vi "data_distributor.vi"(0 "Analog Data Array":T2[](array[typedef]), 1 "Pressure/Temperature/Mixture Properties Refnum":refnum<vi>, 2 "Measurements Data Refnum":refnum<vi>, 3 "Cluster 2":T1, 9 "Indicies":T3[](array[typedef]), 11 "error in":errorcluster, 12 "Diode ChartsRefnum":refnum<vi>, 13 "Vapor PID Refnum":refnum<vi>, 14 "Liquid PID Refnum":refnum<vi>) -> (15 "error out":errorcluster)   [LabVIEW 2017]
uses:
  Utility Sub VIs/pressure_temp_mixture.ctl
  Utility Sub VIs/pulse_generator_data.ctl
  Utility Sub VIs/diode_charts.ctl
  analog_data.ctl
  index_array_cluster.ctl
  Utility Sub VIs/valve_pid_control.ctl
panel:
  # "Pulse Gen"
  # "Test Section"
  # "Saturation\nPressure [Pa]"
  # "Saturation\nTemperature [C]"
  # "Pressure [Pa]"
  # "Temperature [C]"
  # "Liquid Tank"
  # "Separator"
  # "Liquid Inlet"
  # "Vapor Tank"
  # "Vapor Inlet"
  # "Test Section"
  # "Upper Dev Section"
  # "Lower Dev Section"
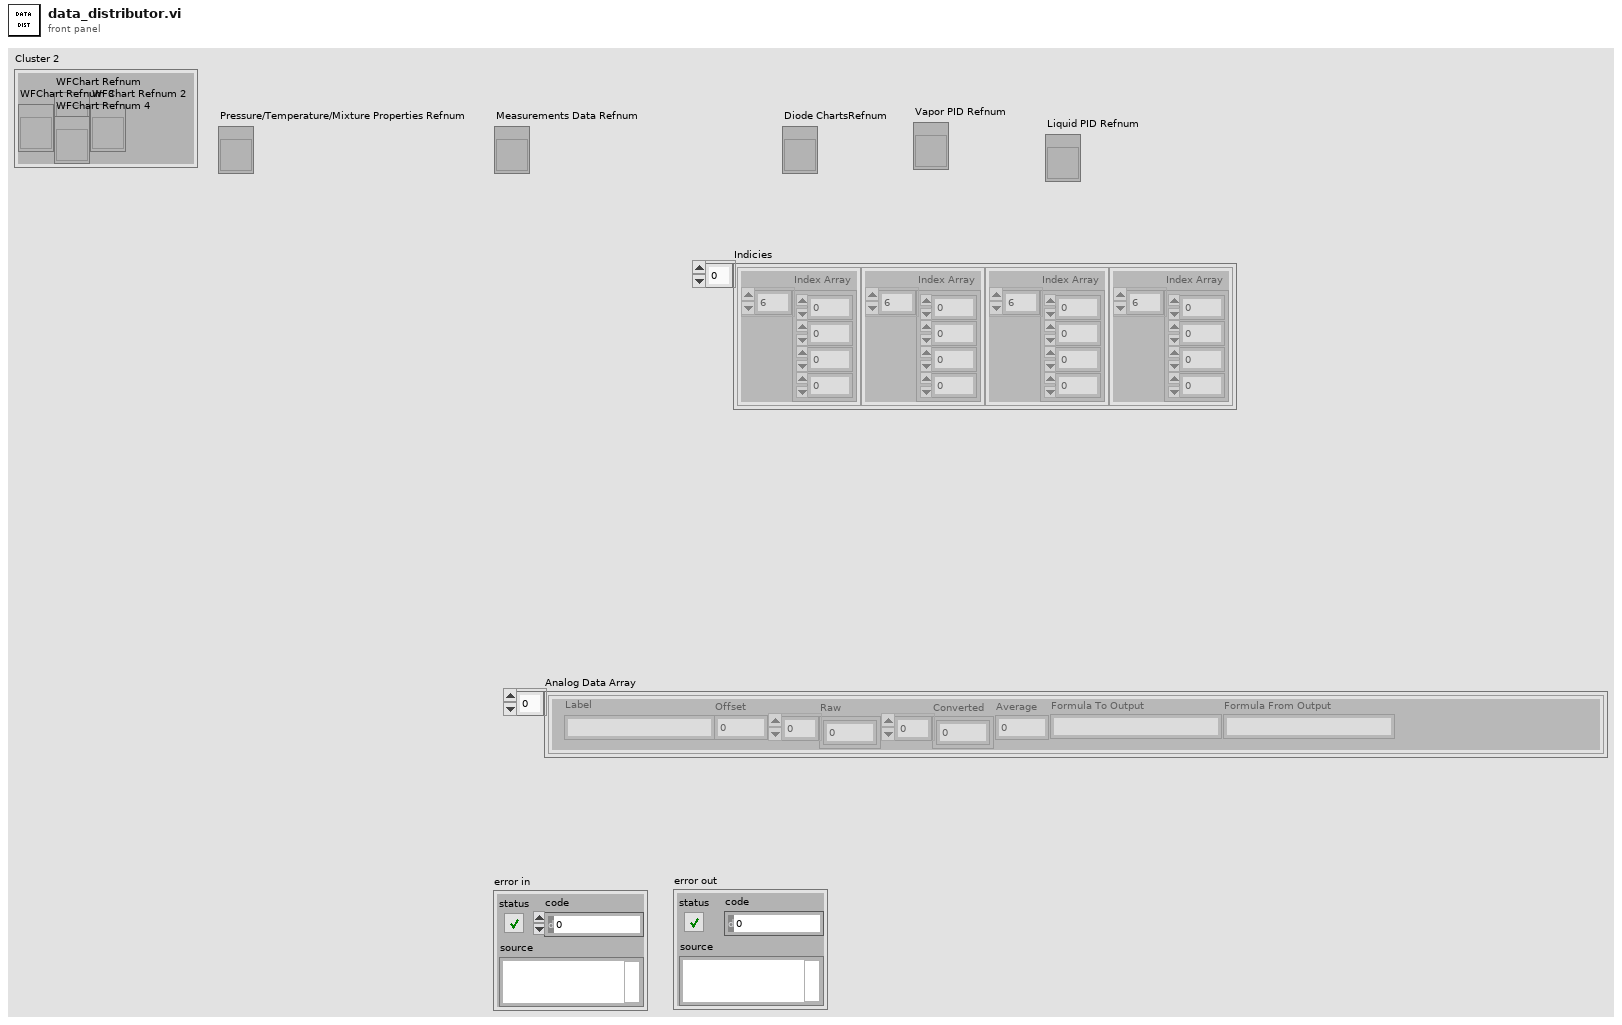
[diagram p1: front panel]
types:
  T1 = cluster{"WFChart Refnum":refnum<vi>, "WFChart Refnum 2":refnum<vi>, "WFChart Refnum 3":refnum<vi>, "WFChart Refnum 4":refnum<vi>}
  T2 = typedef "analog_data.ctl" = cluster{"Label":string, "Offset":dbl, "Raw":dbl[], "Converted":dbl[], "Average":dbl, "Formula To Output":string, "Formula From Output":string}
  T3 = typedef "index_array_cluster.ctl" = cluster{"Index Array":i32[]}
  T4 = cluster{"Mixing Tee dP":dbl, "PG inlet-Mixing Tee Abs Pressure":dbl, "PG inlet-Mixing Tee Temperature":dbl}
  T5 = typedef "pressure_temp_mixture.ctl" = cluster{"Line Densities\n[g/cm^3]":cluster{"Vapor Line":dbl, "Liquid Line":dbl}, "Mixture Properties":cluster{"Enthalpy":dbl, "Quality [-]":dbl}, "Component PTs":cluster{"Liquid Tank P":dbl, "Liquid Tank T":dbl, "Liquid Tank Sat P":dbl, "Liquid Tank Sat T":dbl, "Separator P":dbl, "Separator T":dbl, "Separator Sat P":dbl, "Separator Sat T":dbl, "Liquid Inlet P":dbl, "Liquid Inlet T":dbl, "Liquid Inlet Sat P":dbl, "Liquid Inlet Sat T":dbl, "Vapor Tank P":dbl, "Vapor Tank T":dbl, "Vapor Tank Sat P":dbl, "Vapor Tank Sat T":dbl, "Vapor Inlet P":dbl, "Vapor Inlet T":dbl, "Vapor Inlet Sat P":dbl, "Vapor Inlet Sat T":dbl, "Test Section P":dbl, "Test Section T":dbl, "Test Section Sat P":dbl, "Test Section Sat T":dbl, "Upper Dev Section P":dbl, "Upper Dev Section T":dbl, "Upper Dev Section Sat P":dbl, "Upper Dev Section Sat T":dbl, "Lower Dev Section P":dbl, "Lower Dev Section T":dbl, "Lower Dev Section Sat P":dbl, "Lower Dev Section Sat T":dbl}, "Ambient Pressure [Pa]":dbl, "Mixing Tee":cluster{"Venturi dP":dbl, "PGminiPressure":dbl, "PGminiTemperature":dbl}}
  T6 = cluster{"[0]":dbl, "[1]":dbl, "[2]":dbl, "[3]":dbl, "[4]":dbl, "[5]":dbl, "[6]":dbl, "[7]":dbl, "[8]":dbl, "[9]":dbl, "[10]":dbl, "[11]":dbl, "[12]":dbl, "[13]":dbl, "[14]":dbl, "[15]":dbl, "[16]":dbl, "[17]":dbl, "[18]":dbl, "[19]":dbl, "[20]":dbl, "[21]":dbl, "[22]":dbl, "[23]":dbl, "[24]":dbl, "[25]":dbl, "[26]":dbl, "[27]":dbl, "[28]":dbl, "[29]":dbl, "[30]":dbl, "[31]":dbl}
  T7 = cluster{"Mass Flow Rate [g/s]":dbl, "Mass Flow Rate [g/s]":dbl}
  T8 = cluster{"[0]":dbl, "[1]":dbl, "[2]":dbl, "[3]":dbl, "[4]":dbl, "[5]":dbl, "[6]":dbl, "[7]":dbl, "[8]":dbl, "[9]":dbl, "[10]":dbl, "[11]":dbl, "[12]":dbl, "[13]":dbl, "[14]":dbl, "[15]":dbl}
  T9 = typedef "valve_pid_control.ctl" = cluster{"Flow":cluster{"Flow rate [g/s]":dbl, "Line Density [g/cm^3]":dbl}, "Valve On/Off":bool, "PID Mode":bool, "PLC Calc Basis":bool, "Flow Set Point [g/s]":dbl, "Pump Output [%]":dbl, "Valve Open Voltage [V]":dbl, "Flow Setpoint Adrs":u16, "Pump Output Adrs":u16, "Manual Mode Request Adrs":u16, "Manual Mode Adrs":u16}
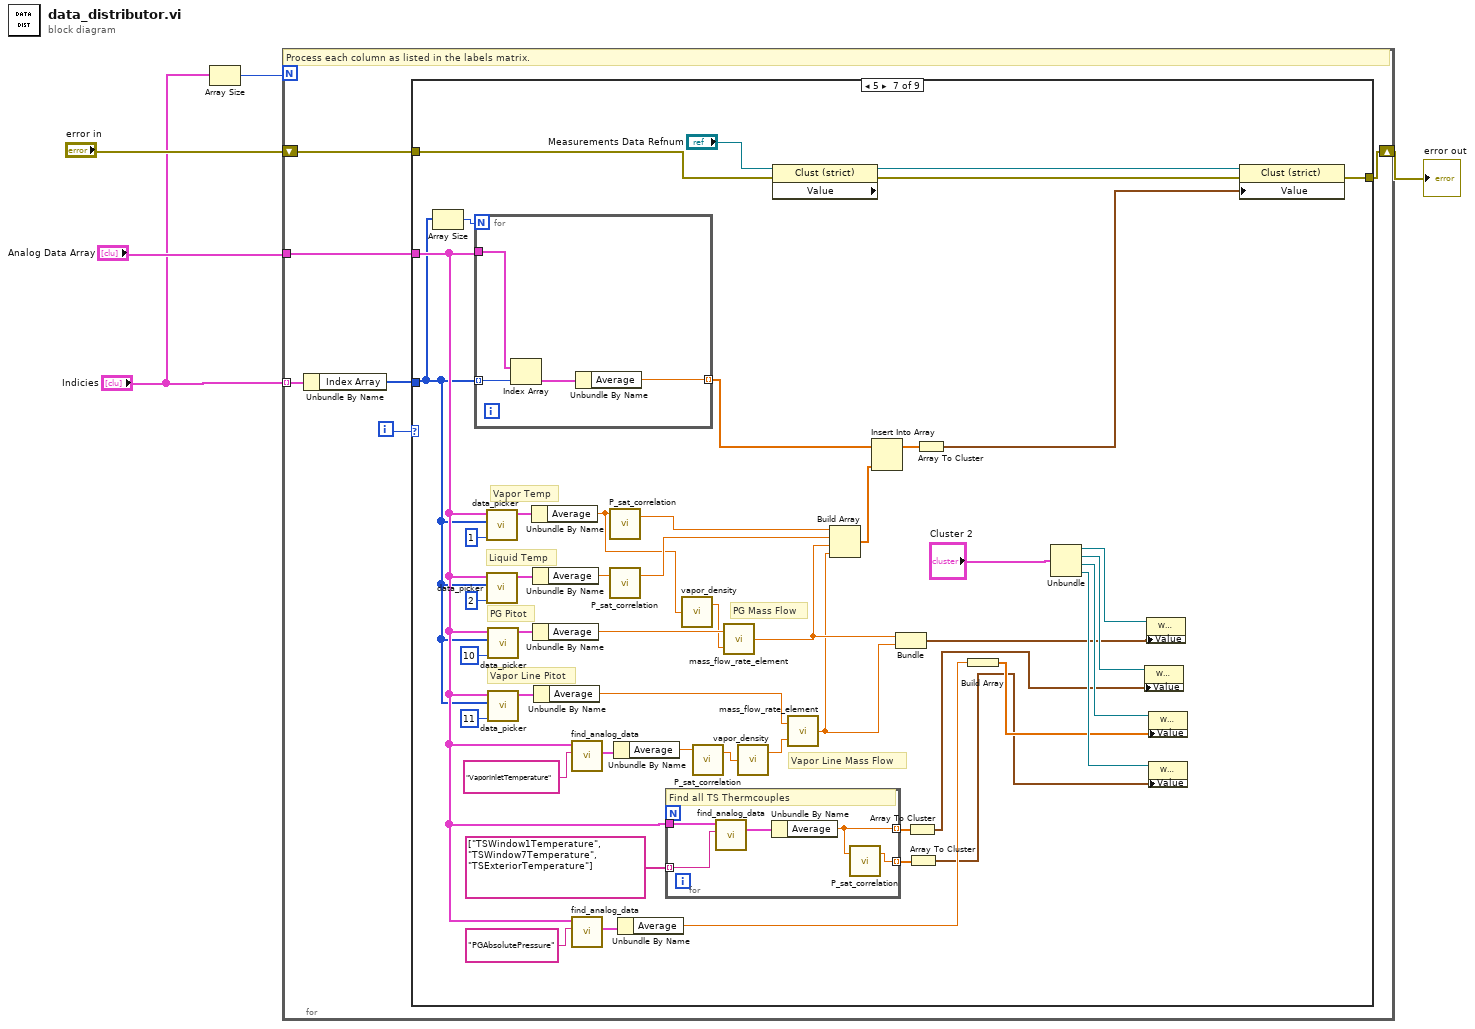
[diagram p0: block diagram]
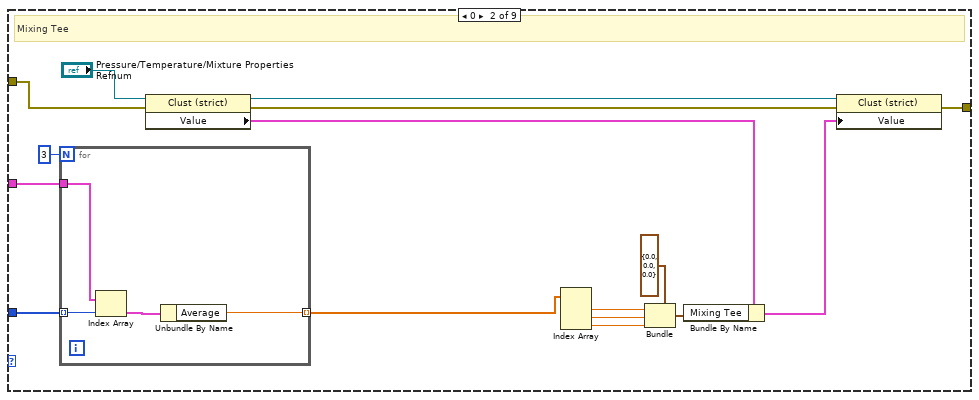
[diagram p3: hidden frame]
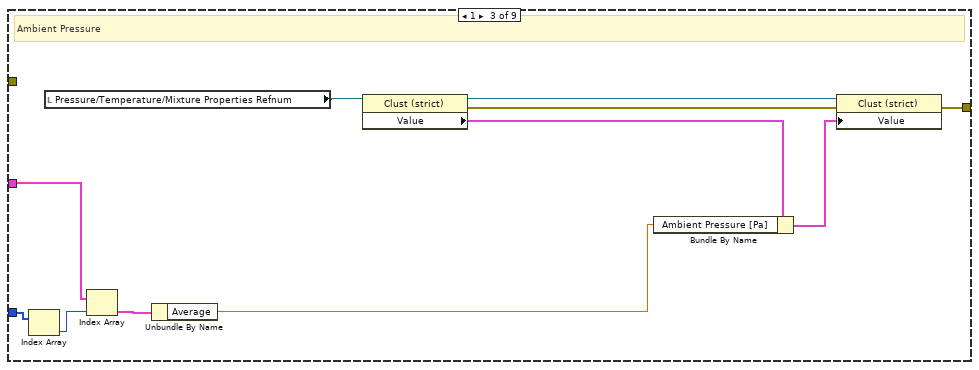
[diagram p4: hidden frame]
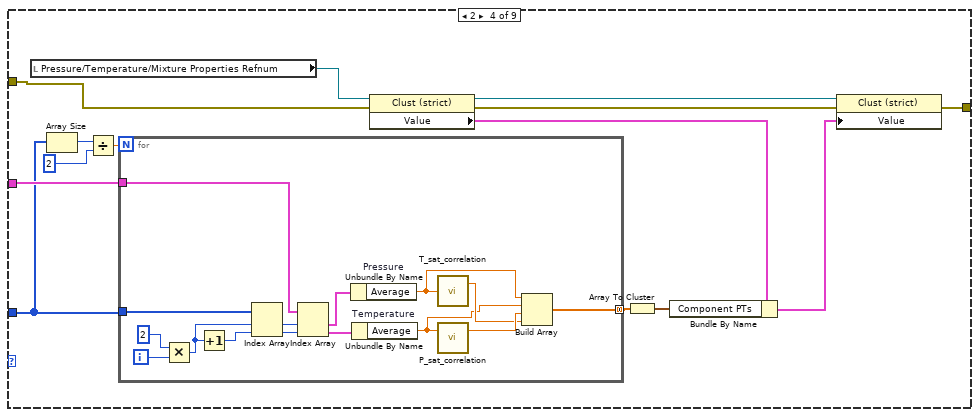
[diagram p5: hidden frame]
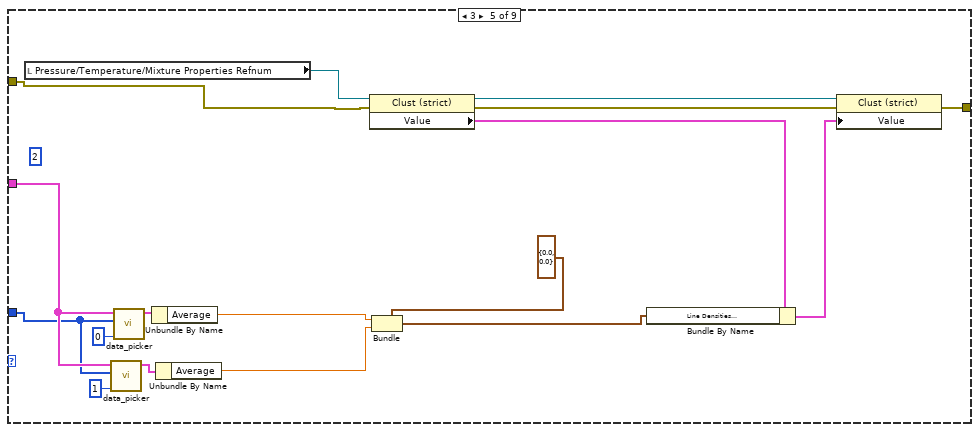
[diagram p6: hidden frame]
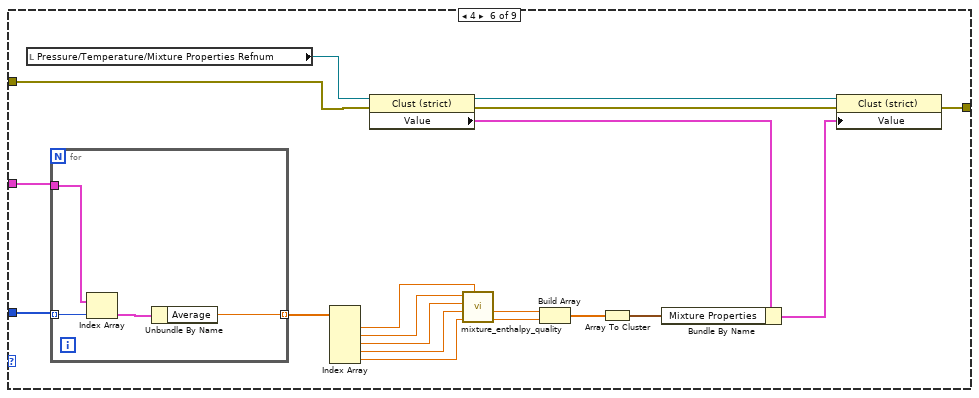
[diagram p7: hidden frame]
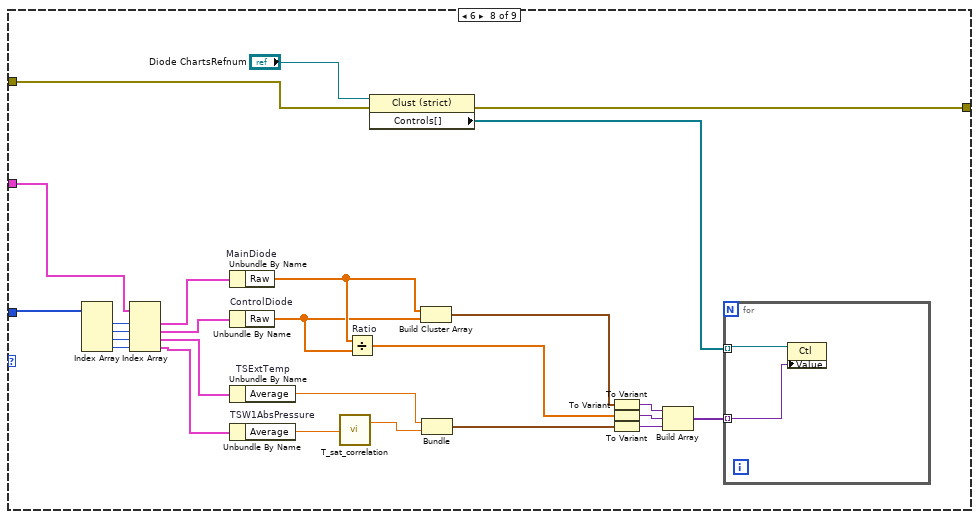
[diagram p8: hidden frame]
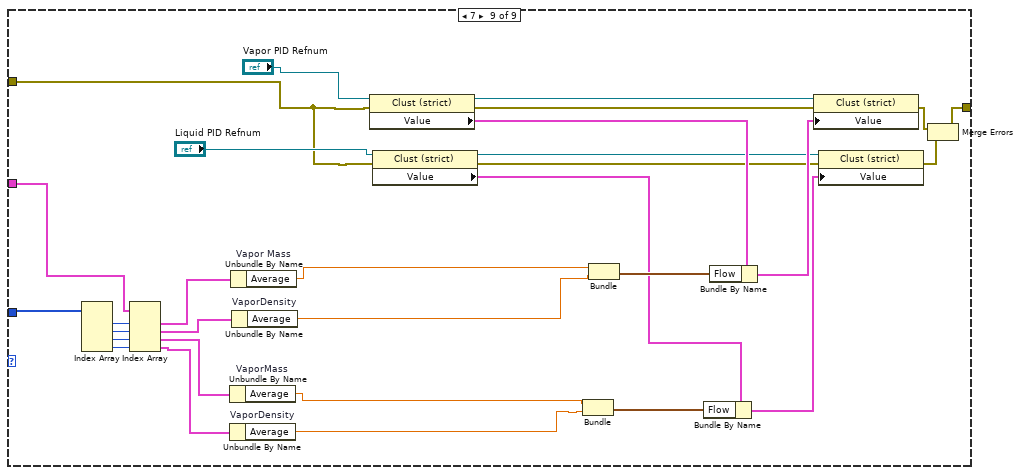
[diagram p9: hidden frame]
diagram:
  n1 = Array Size(array="Indicies") -> (size(s)=w4:i32)
  n2 = for {
    N: w4 -> [_]
    tunnel: "Analog Data Array" -> [w10]
    tunnel: "Indicies" -> [w6] mode=indexing
    shift-right: [w8] -> w5
    shift-left: "error in" -> [w9]
    i -> [w11]
    # "Process each column as listed in the labels matrix."
    n3 = Unbundle By Name(w6) -> ("Index Array"=w7:i32[])
    n4 = case shown="5" w11 {
      tunnel: w7 -> [_ w24 w34 w52 w79 w103 w122 w191 w228]
      tunnel: w10 -> [_ w23 w39 w53 w80 w104 w130 w189 w226]
      tunnel: w9 -> [w12 w20 _ w44 w84 w91 w124 w171 w200]
      tunnel: [w12 w22 w37 w46 w85 w92 w127 w173 w202] -> w8
      frame Default {
      }
      frame 0 {
        # "Mixing Tee"
        n5 = for {
          N: 3 -> [_]
          tunnel: w24 -> [w32] mode=indexing
          tunnel: w23 -> [w31]
          tunnel: [w29] -> w17 mode=indexing
          n6 = Index Array(array=w31, index=w32) -> (element=w30:T2)
          n7 = Unbundle By Name(w30) -> ("Average"=w29:dbl)
        }
        n8 = property class="Clust (strict)"(reference="Pressure/Temperature/Mixture Properties Refnum", error in=w20) -> (reference out=w25:refnum<vi>, error out=w26:errorcluster, "Value"=w28:T5)
        n9 = Index Array(array=w17) -> (element #1=w15:dbl, element #2=w14:dbl, element #3=w13:dbl)  [unwired: 3 in]
        n10 = Bundle(cluster=T4 {"Mixing Tee dP"=0.0, "PG inlet-Mixing Tee Abs Pressure"=0.0, "PG inlet-Mixing Tee Temperature"=0.0} ("Mixing Tee"), "Mixing Tee dP"=w15, "PG inlet-Mixing Tee Abs Pressure"=w14, "PG inlet-Mixing Tee Temperature"=w13) -> (w19:T4)
        n11 = Bundle By Name(cluster=w28, "Mixing Tee"=w19) -> (w27:T5)
        n12 = property class="Clust (strict)"(reference=w25, error in=w26, "Value"=w27) -> (error out=w22:errorcluster)  [unwired: 1 out]
      }
      frame 1 {
        # "Ambient Pressure"
        n13 = Index Array(array=w34) -> (element=w33:i32)  [unwired: 1 in]
        n14 = local read "Pressure/Temperature/Mixture Properties Refnum"() -> (w36:refnum<vi>)
        n15 = Index Array(array=w39, index=w33) -> (element=w35:T2)
        n16 = Unbundle By Name(w35) -> ("Average"=w38:dbl)
        n17 = property class="Clust (strict)"(reference=w36) -> (reference out=w40:refnum<vi>, error out=w41:errorcluster, "Value"=w43:T5)  [unwired: 1 in]
        n18 = Bundle By Name(cluster=w43, "Ambient Pressure [Pa]"=w38) -> (w42:T5)
        n19 = property class="Clust (strict)"(reference=w40, error in=w41, "Value"=w42) -> (error out=w37:errorcluster)  [unwired: 1 out]
      }
      frame 2 {
        n20 = local read "Pressure/Temperature/Mixture Properties Refnum"() -> (w45:refnum<vi>)
        n21 = Array Size(array=w52) -> (size(s)=w50:i32)
        n22 = Divide(x=w50, y=2) -> (x/y=w51:dbl)
        n23 = for {
          N: w51 -> [_]
          tunnel: w52 -> [w68]
          tunnel: w53 -> [w72]
          tunnel: [w58] -> w48 mode=concatenating
          i -> [w70]
          n24 = Multiply(x=2, y=w70) -> (x*y=w66:i32)
          n25 = Increment(x=w66) -> (x+1=w67:i32)
          n26 = Index Array(array=w68, index #1=w66, index #2=w67) -> (element #1=w65:i32, element #2=w64:i32)
          n27 = Index Array(array=w72, index #1=w65, index #2=w64) -> (element #1=w71:T2, element #2=w63:T2)
          n28 = Unbundle By Name "Pressure"(w71) -> ("Average"=w60:dbl)
          n29 = Unbundle By Name "Temperature"(w63) -> ("Average"=w59:dbl)
          n30 = call "T_sat_correlation.vi"("P [Pa]"=w60) -> ("T Sat [C]"=w61:dbl)  [unwired: 1 out]
          n31 = call "P_sat_correlation.vi"("Temperature[C]"=w59) -> ("P Sat[Pa]"=w62:dbl)  [unwired: 1 in, 1 out]
          n32 = Build Array(w60, w59, w62, w61) -> (w58:dbl[])
        }
        n33 = property class="Clust (strict)"(reference=w45, error in=w44) -> (reference out=w54:refnum<vi>, error out=w55:errorcluster, "Value"=w57:T5)
        n34 = Array To Cluster(array=w48) -> (cluster=w47:T6)
        n35 = Bundle By Name(cluster=w57, "Component PTs"=w47) -> (w56:T5)
        n36 = property class="Clust (strict)"(reference=w54, error in=w55, "Value"=w56) -> (error out=w46:errorcluster)  [unwired: 1 out]
      }
      frame 3 {
        (unwired) 2
        n37 = local read "Pressure/Temperature/Mixture Properties Refnum"() -> (w83:refnum<vi>)
        n38 = call "data_picker.vi"("index"=1, "Indicies"=w79, "Data in"=w80) -> ("Data Out"=w77:T2)  [unwired: 8 in]
        n39 = call "data_picker.vi"("index"=0, "Indicies"=w79, "Data in"=w80) -> ("Data Out"=w82:T2)  [unwired: 8 in]
        n40 = Unbundle By Name(w82) -> ("Average"=w74:dbl)
        n41 = Unbundle By Name(w77) -> ("Average"=w73:dbl)
        n42 = property class="Clust (strict)"(reference=w83, error in=w84) -> (reference out=w86:refnum<vi>, error out=w87:errorcluster, "Value"=w89:T5)
        n43 = Bundle(cluster=cluster{"[0]":dbl, "[1]":dbl} {"[0]"=0.0, "[1]"=0.0}, "[0]"=w74, "[1]"=w73) -> (w75:cluster{"[0]":dbl, "[1]":dbl})
        n44 = Bundle By Name(cluster=w89, "Line Densities\n[g/cm^3]"=w75) -> (w88:T5)
        n45 = property class="Clust (strict)"(reference=w86, error in=w87, "Value"=w88) -> (error out=w85:errorcluster)  [unwired: 1 out]
      }
      frame 4 {
        n46 = local read "Pressure/Temperature/Mixture Properties Refnum"() -> (w90:refnum<vi>)
        n47 = for {
          tunnel: w103 -> [w112] mode=indexing
          tunnel: w104 -> [w111]
          tunnel: [w109] -> w102 mode=indexing
          n48 = Index Array(array=w111, index=w112) -> (element=w110:T2)
          n49 = Unbundle By Name(w110) -> ("Average"=w109:dbl)
        }
        n50 = Index Array(array=w102) -> (element #1=w97:dbl, element #2=w96:dbl, element #3=w95:dbl, element #4=w94:dbl, element #5=w93:dbl)  [unwired: 5 in]
        n51 = property class="Clust (strict)"(reference=w90, error in=w91) -> (reference out=w105:refnum<vi>, error out=w106:errorcluster, "Value"=w108:T5)
        n52 = call "mixture_enthalpy_quality.vi"("Vapor Inlet Pressure [Pa]"=w97, "Separator Temp [C]"=w93, "Liquid Inlet Temp [C]"=w94, "Vapor Flow Rate [g/s]"=w95, "Liquid Flow Rate [g/s]"=w96) -> ("Quality [-]"=w100:dbl, "mixture enthalpy"=w101:dbl)  [unwired: 2 out]
        n53 = Build Array(w101, w100) -> (w99:dbl[])
        n54 = Array To Cluster(array=w99) -> (cluster=w98:cluster{"[0]":dbl, "[1]":dbl})
        n55 = Bundle By Name(cluster=w108, "Mixture Properties"=w98) -> (w107:T5)
        n56 = property class="Clust (strict)"(reference=w105, error in=w106, "Value"=w107) -> (error out=w92:errorcluster)  [unwired: 1 out]
      }
      frame 5 {
        # "Vapor Line Mass Flow"
        # "PG Mass Flow"
        # "PG Pitot"
        # "Vapor Line Pitot"
        # "Liquid Temp"
        # "Vapor Temp"
        n57 = Array Size(array=w122) -> (size(s)=w123:i32)
        n58 = for {
          N: w123 -> [_]
          tunnel: w122 -> [w170] mode=indexing
          tunnel: w130 -> [w169]
          tunnel: [w167] -> w143 mode=indexing
          n59 = Index Array(array=w169, index=w170) -> (element=w168:T2)
          n60 = Unbundle By Name(w168) -> ("Average"=w167:dbl)
        }
        n61 = call "data_picker.vi"("index"=1, "Indicies"=w122, "Data in"=w130) -> ("Data Out"=w137:T2)  [unwired: 8 in]
        n62 = call "data_picker.vi"("index"=2, "Indicies"=w122, "Data in"=w130) -> ("Data Out"=w157:T2)  [unwired: 8 in]
        n63 = call "data_picker.vi"("index"=10, "Indicies"=w122, "Data in"=w130) -> ("Data Out"=w154:T2)  [unwired: 8 in]
        n64 = call "data_picker.vi"("index"=11, "Indicies"=w122, "Data in"=w130) -> ("Data Out"=w155:T2)  [unwired: 8 in]
        n65 = Unbundle By Name(w137) -> ("Average"=w126:dbl)
        n66 = Unbundle By Name(w157) -> ("Average"=w156:dbl)
        n67 = Unbundle By Name(w154) -> ("Average"=w151:dbl)
        n68 = Unbundle By Name(w155) -> ("Average"=w144:dbl)
        n69 = call "find_analog_data.vi"("Needle"="VaporInletTemperature", "Haystack"=w130) -> ("Needle Out"=w148:T2)  [unwired: 7 in, 2 out]
        n70 = call "find_analog_data.vi"("Needle"="PGAbsolutePressure", "Haystack"=w130) -> ("Needle Out"=w135:T2)  [unwired: 7 in, 2 out]
        n71 = call "P_sat_correlation.vi"("Temperature[C]"=w126) -> ("P Sat[Pa]"=w142:dbl)  [unwired: 1 in, 1 out]
        n72 = call "P_sat_correlation.vi"("Temperature[C]"=w156) -> ("P Sat[Pa]"=w141:dbl)  [unwired: 1 in, 1 out]
        n73 = Unbundle By Name(w148) -> ("Average"=w147:dbl)
        n74 = Unbundle By Name(w135) -> ("Average"=w134:dbl)
        n75 = for {
          tunnel: string[] ["TSWindow1Temperature", "TSWindow7Temperature", "TSExteriorTemperature"] ("Needle") -> [w165] mode=indexing
          tunnel: w130 -> [w166]
          tunnel: [w163] -> w129 mode=indexing
          tunnel: [w162] -> w128 mode=indexing
          # "Find all TS Thermcouples"
          n76 = call "find_analog_data.vi"("Needle"=w165, "Haystack"=w166) -> ("Needle Out"=w164:T2)  [unwired: 7 in, 2 out]
          n77 = Unbundle By Name(w164) -> ("Average"=w163:dbl)
          n78 = call "P_sat_correlation.vi"("Temperature[C]"=w163) -> ("P Sat[Pa]"=w162:dbl)  [unwired: 1 in, 1 out]
        }
        n79 = call "vapor_density.vi"("Vapor Temp [C]"=w126) -> ("Vapor Density[g/cm3]"=w150:dbl)  [unwired: 1 out]
        n80 = call "P_sat_correlation.vi"("Temperature[C]"=w147) -> ("P Sat[Pa]"=w146:dbl)  [unwired: 1 in, 1 out]
        n81 = call "mass_flow_rate_element.vi"("Density [g/cm3]"=w150, "dP [Pa]"=w151) -> ("Mass Flow Rate [g/s]"=w133:dbl)
        n82 = call "vapor_density.vi"("Vapor Temp [C]"=w146) -> ("Vapor Density[g/cm3]"=w145:dbl)  [unwired: 1 out]
        n83 = property class="Clust (strict)" props=["Value"](reference="Measurements Data Refnum", error in=w124) -> (reference out=w160:refnum<vi>, error out=w161:errorcluster)  [unwired: 1 out]
        n84 = call "mass_flow_rate_element.vi"("Density [g/cm3]"=w145, "dP [Pa]"=w144) -> ("Mass Flow Rate [g/s]"=w132:dbl)
        n85 = Build Array(w142, w141, w133, w132) -> (w140:dbl[])
        n86 = Insert Into Array(array=w143, new element=w140) -> (w139:dbl[])  [unwired: 1 in]
        n87 = Bundle("Mass Flow Rate [g/s]"=w133, "Mass Flow Rate [g/s]"=w132) -> (w116:T7)  [unwired: 1 in]
        n88 = Array To Cluster(array=w129) -> (cluster=w115:cluster{"[0]":dbl, "[1]":dbl, "[2]":dbl})
        n89 = Array To Cluster(array=w128) -> (cluster=w113:cluster{"[0]":dbl, "[1]":dbl})
        n90 = Array To Cluster(array=w139) -> (cluster=w138:T8)
        n91 = Build Array(w134) -> (w114:dbl[])
        n92 = Unbundle("Cluster 2") -> ("WFChart Refnum"=w120:refnum<vi>, "WFChart Refnum 2"=w119:refnum<vi>, "WFChart Refnum 3"=w118:refnum<vi>, "WFChart Refnum 4"=w117:refnum<vi>)
        n93 = property class="WFChart (strict)"(reference=w119, "Value"=w115) -> ()  [unwired: 1 in, 2 out]
        n94 = property class="WFChart (strict)"(reference=w120, "Value"=w116) -> ()  [unwired: 1 in, 2 out]
        n95 = property class="WFChart (strict)"(reference=w118, "Value"=w114) -> ()  [unwired: 1 in, 2 out]
        n96 = property class="WFChart (strict)"(reference=w117, "Value"=w113) -> ()  [unwired: 1 in, 2 out]
        n97 = property class="Clust (strict)"(reference=w160, error in=w161, "Value"=w138) -> (error out=w127:errorcluster)  [unwired: 1 out]
      }
      frame 6 {
        n98 = Index Array(array=w191) -> (element #1=w186:i32, element #2=w190:i32, element #3=w188:i32, element #4=w187:i32)  [unwired: 4 in]
        n99 = Index Array(array=w189, index #1=w186, index #2=w190, index #3=w188, index #4=w187) -> (element #1=w185:T2, element #2=w184:T2, element #3=w179:T2, element #4=w178:T2)
        n100 = Unbundle By Name "MainDiode"(w185) -> ("Raw"=w183:dbl[])
        n101 = Unbundle By Name "ControlDiode"(w184) -> ("Raw"=w182:dbl[])
        n102 = Unbundle By Name "TSExtTemp"(w179) -> ("Average"=w176:dbl)
        n103 = Unbundle By Name "TSW1AbsPressure"(w178) -> ("Average"=w177:dbl)
        n104 = call "T_sat_correlation.vi"("P [Pa]"=w177) -> ("T Sat [C]"=w175:dbl)  [unwired: 1 out]
        n105 = Divide "Ratio"(x=w183, y=w182) -> (x/y=w180:dbl[])
        n106 = property class="Clust (strict)"(reference="Diode ChartsRefnum", error in=w171) -> (error out=w173:errorcluster, "Controls[]"=w192:refnum<vi>[])  [unwired: 1 out]
        n107 = Build Cluster Array(w183, w182) -> (w181:cluster{dbl, dbl}[])
        n108 = Bundle("Average"=w176, "T Sat [C]"=w175) -> (w174:cluster{"Average":dbl, "T Sat [C]":dbl})  [unwired: 1 in]
        n109 = To Variant(anything=w181) -> (Variant=w196:variant)
        n110 = To Variant(anything=w180) -> (Variant=w195:variant)
        n111 = To Variant(anything=w174) -> (Variant=w194:variant)
        n112 = Build Array(w196, w195, w194) -> (w193:variant[])
        n113 = for {
          tunnel: w192 -> [w198] mode=indexing
          tunnel: w193 -> [w197] mode=indexing
          n114 = property class="Ctl"(reference=w198, "Value"=w197) -> ()  [unwired: 1 in, 2 out]
        }
      }
      frame 7 {
        n115 = Index Array(array=w228) -> (element #1=w223:i32, element #2=w227:i32, element #3=w225:i32, element #4=w224:i32)  [unwired: 4 in]
        n116 = Index Array(array=w226, index #1=w223, index #2=w227, index #3=w225, index #4=w224) -> (element #1=w222:T2, element #2=w221:T2, element #3=w220:T2, element #4=w219:T2)
        n117 = Unbundle By Name "VaporMass"(w220) -> ("Average"=w210:dbl)
        n118 = Unbundle By Name "VaporDensity"(w219) -> ("Average"=w209:dbl)
        n119 = Unbundle By Name "Vapor Mass"(w222) -> ("Average"=w217:dbl)
        n120 = Unbundle By Name "VaporDensity"(w221) -> ("Average"=w216:dbl)
        n121 = property class="Clust (strict)"(reference="Vapor PID Refnum", error in=w200) -> (reference out=w214:refnum<vi>, error out=w213:errorcluster, "Value"=w218:T9)
        n122 = property class="Clust (strict)"(reference="Liquid PID Refnum", error in=w200) -> (reference out=w208:refnum<vi>, error out=w207:errorcluster, "Value"=w206:T9)
        n123 = Bundle("Average"=w210, "Average"=w209) -> (w211:cluster{"Average":dbl, "Average":dbl})  [unwired: 1 in]
        n124 = Bundle("Average"=w217, "Average"=w216) -> (w215:cluster{"Average":dbl, "Average":dbl})  [unwired: 1 in]
        n125 = Bundle By Name(cluster=w206, "Flow"=w211) -> (w205:T9)
        n126 = Bundle By Name(cluster=w218, "Flow"=w215) -> (w212:T9)
        n127 = property class="Clust (strict)"(reference=w214, error in=w213, "Value"=w212) -> (error out=w204:errorcluster)  [unwired: 1 out]
        n128 = property class="Clust (strict)"(reference=w208, error in=w207, "Value"=w205) -> (error out=w203:errorcluster)  [unwired: 1 out]
        n129 = Merge Errors(w204, w203) -> (w202:errorcluster)
      }
    }
  }
  "error out" <- w5
